vi "KB-4PointtoFlatness.vi"(10 "Src Data":dbl[][](array[numeric]), 11 "矩形ROS":string[](array[string])) -> (3 "bASER":cluster{"X":i32, "Y":i32, "Z":dbl}[](array[cluster]))   [LabVIEW 2015]
panel:
  out "bottom":i32
  out "Right":i32
  out "Top":i32
  out "Left":i32
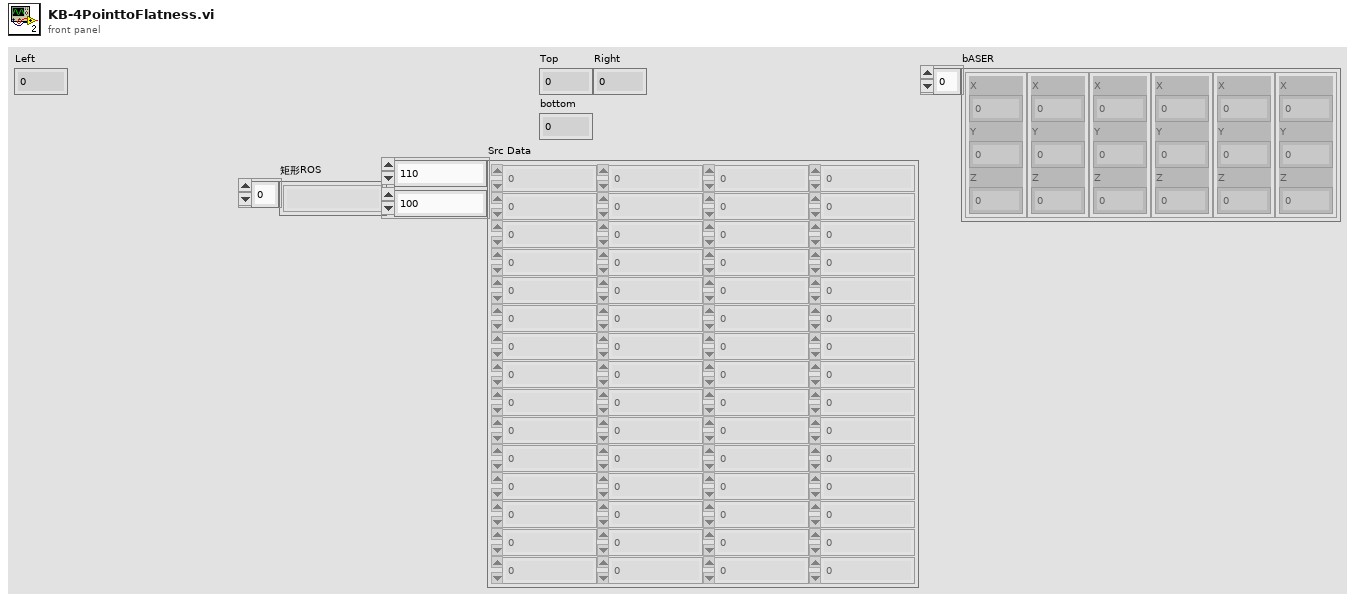
[diagram p1: front panel]
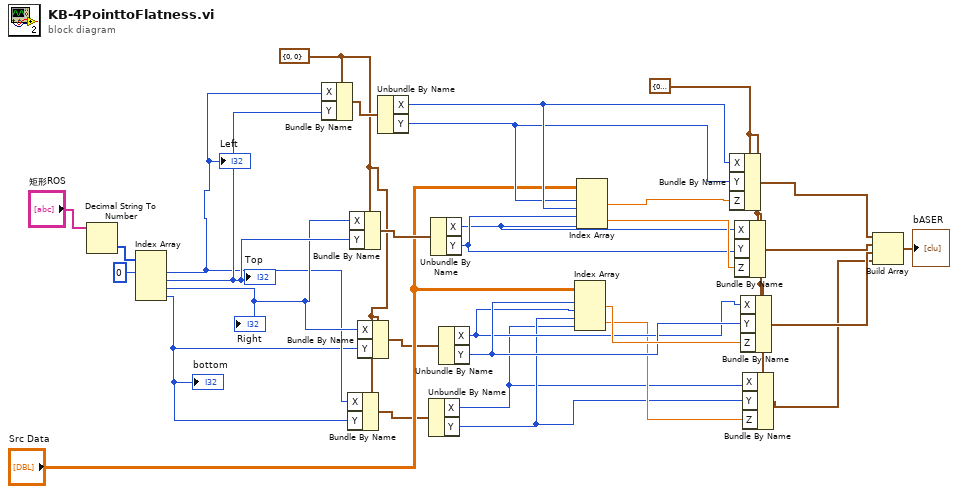
[diagram p0: block diagram]
diagram:
  w13 = cluster{"X":i32, "Y":i32, "Z":dbl} {"X"=0, "Y"=0, "Z"=0.0}
  w14 = cluster{"X":i32, "Y":i32} {"X"=0, "Y"=0}
  n1 = Decimal String To Number(string="矩形ROS") -> (number=w30:i32[])  [unwired: 2 in, 1 out]
  n2 = Index Array(array=w30, index #1=0 ("索引")) -> (element #1=w2:i32, element #2=w4:i32, element #3=w3:i32, element #4=w1:i32)  [unwired: 3 in]
  "Left" <- w2
  "Top" <- w4
  "Right" <- w3
  "bottom" <- w1
  n3 = Bundle By Name(cluster=w14, "X"=w2, "Y"=w4) -> (w28:cluster{"X":i32, "Y":i32})
  n4 = Bundle By Name(cluster=w14, "X"=w2, "Y"=w1) -> (w15:cluster{"X":i32, "Y":i32})
  n5 = Bundle By Name(cluster=w14, "X"=w3, "Y"=w4) -> (w24:cluster{"X":i32, "Y":i32})
  n6 = Bundle By Name(cluster=w14, "X"=w3, "Y"=w1) -> (w19:cluster{"X":i32, "Y":i32})
  n7 = Unbundle By Name(w28) -> ("X"=w26:i32, "Y"=w25:i32)
  n8 = Unbundle By Name(w15) -> ("X"=w10:i32, "Y"=w11:i32)
  n9 = Unbundle By Name(w24) -> ("X"=w21:i32, "Y"=w22:i32)
  n10 = Unbundle By Name(w19) -> ("X"=w16:i32, "Y"=w17:i32)
  n11 = Index Array(array="Src Data", index (row) #1=w17, index (col) #1=w16, index (row) #2=w11, index (col) #2=w10) -> (element #1=w18:dbl, element #2=w12:dbl)
  n12 = Index Array(array="Src Data", index (row) #1=w25, index (col) #1=w26, index (row) #2=w22, index (col) #2=w21) -> (element #1=w27:dbl, element #2=w23:dbl)
  n13 = Bundle By Name(cluster=w13, "X"=w26, "Y"=w25, "Z"=w27) -> (w9:cluster{"X":i32, "Y":i32, "Z":dbl})
  n14 = Bundle By Name(cluster=w13, "X"=w21, "Y"=w22, "Z"=w23) -> (w8:cluster{"X":i32, "Y":i32, "Z":dbl})
  n15 = Bundle By Name(cluster=w13, "X"=w16, "Y"=w17, "Z"=w18) -> (w7:cluster{"X":i32, "Y":i32, "Z":dbl})
  n16 = Bundle By Name(cluster=w13, "X"=w10, "Y"=w11, "Z"=w12) -> (w6:cluster{"X":i32, "Y":i32, "Z":dbl})
  n17 = Build Array(w9, w8, w7, w6) -> (→"bASER":cluster{"X":i32, "Y":i32, "Z":dbl}[])
